vi "Write Sine Wave.vi"(8 "error in (no error)":errorcluster, 10 "Sin Wave Parameters":T1={"phase"=0.0, "amplitude"=1.0, "frequency"=10.0, "offset"=0.0} {"offset" format="%#_13g"; "frequency" format="%0.2p"; "amplitude" format="%0.2p"; "phase" format="%.2p"}, 11 "Analog Output Channel in":refnum<class "Analog Output Channel.lvclass">) -> (0 "error out":errorcluster, 3 "Analog Output Channel out":refnum<class "Analog Output Channel.lvclass">)   [LabVIEW 2015, in "Analog Output Channel.lvlib" / "Analog Output Channel.lvclass"]
uses:
  Analog Output Channel.lvclass
  AOChData.lvclass
  <vilib>/measure/NI_MABase.lvlib
  Channel/Channel/Channel.lvclass
panel:
  out "signal out":waveform(dbl)
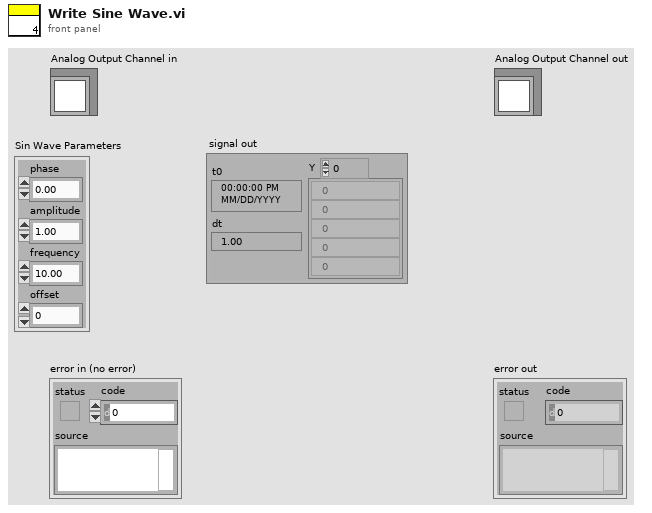
[diagram p1: front panel]
types:
  T1 = cluster{"phase":dbl, "amplitude":dbl, "frequency":dbl, "offset":dbl}
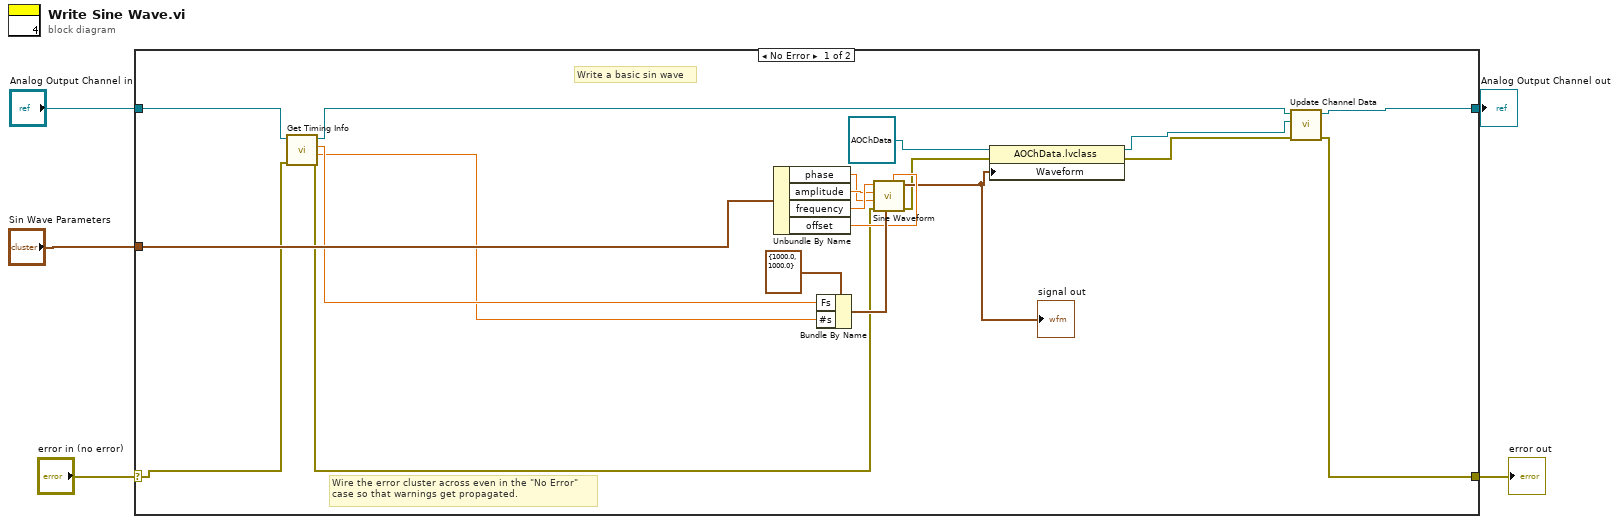
[diagram p0: block diagram]
diagram:
  n1 = case shown="No Error" "error in (no error)" {
    selector: "error in (no error)" -> [w7 w27]
    tunnel: [w12 w27] -> w4
    tunnel: [w16 w26] -> w2
    tunnel: "Analog Output Channel in" -> [w11 w26]
    tunnel: "Sin Wave Parameters" -> [w23 _]
    frame No Error {
      # "Write a basic sin wave"
      # "Wire the error cluster across even in the \"No Error\"\ncase so that warnings get propagated."
      n2 = call "Get Timing Info.vi"("error in (no error)"=w7, "Channel in"=w11) -> ("error out"=w6:errorcluster, "Buffer Size"=w8:dbl, "Sample Rate"=w9:dbl, "Channel out"=w10:refnum<class "Analog Output Channel.lvclass">)  [unwired: 6 in]
      n3 = Unbundle By Name(w23) -> ("phase"=w19:dbl, "amplitude"=w20:dbl, "frequency"=w21:dbl, "offset"=w22:dbl)
      n4 = Bundle By Name(cluster=cluster{"Fs":dbl, "#s":dbl} {"Fs"=1000.0, "#s"=1000.0} ("sampling info"), "Fs"=w9, "#s"=w8) -> (w24:cluster{"Fs":dbl, "#s":dbl})
      n5 = call <vilib>:"Sine Waveform.vi"("offset"=w22, "sampling info"=w24, "error in (no error)"=w6, "phase"=w19, "amplitude"=w20, "frequency"=w21) -> ("error out"=w13:errorcluster, "signal out"=w17:waveform(dbl))  [unwired: 4 in]
      "signal out" <- w17
      n6 = property class="AOChData.lvclass"(reference=refnum<class "AOChData.lvclass"> refnum ("Analog Output Channel.lvlib:AOChData.lvclass"), error in=w13, "Waveform"=w17) -> (reference out=w15:refnum<class "AOChData.lvclass">, error out=w14:errorcluster)
      n7 = call "Update Channel Data.vi"("error in (no error)"=w14, "ChannelData"=w15, "Channel in"=w10) -> ("error out"=w12:errorcluster, "Channel out"=w16:refnum<class "Analog Output Channel.lvclass">)  [unwired: 7 in]
    }
    frame Error {
    }
  }
  "error out" <- w4
  "Analog Output Channel out" <- w2
